vi "RSZVB Set Trace Format ZVR.vi"(8 "error in (no error)":errorcluster {"code" format="%.0x"}, 10 "Data Format (0: Unformatted)":i32(ring) items=["Unformatted", "Formatted", "Unformatted With Trace Mathematics"], 11 "VISA session":refnum<visa-resource-name>) -> (0 "error out":errorcluster {"code" format="%.0x"}, 3 "dup VISA session":refnum<visa-resource-name>)   [LabVIEW 2011]
doc: "This VI defines the format for traces retrieved with the ZVR-compatible command TRACe[:DATA][:RESPonse][:ALL]? \n\nNote(s):\n\n(1) This VI is ZVR compatible.\n\nRemote-control command(s):\nFORMat:DEXPort:SOURce FDATa | SDATa | MDATa"
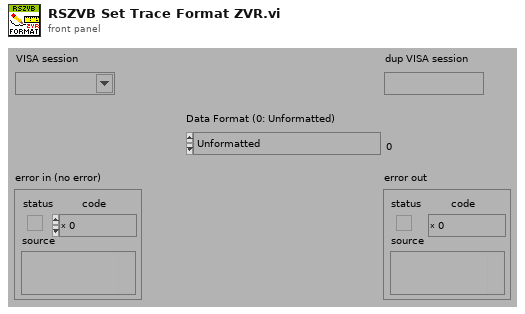
[diagram p1: front panel]
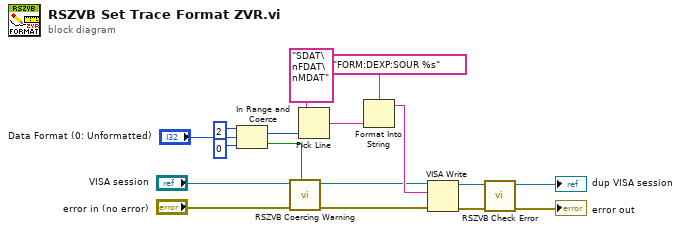
[diagram p0: block diagram]
diagram:
  n1 = In Range and Coerce(upper limit=2, x="Data Format (0: Unformatted)", lower limit=0) -> (coerced(x)=w14:i32, In Range?=w2:bool)
  n2 = call "RSZVB Coercing Warning.vi"("In Range?"=w2, "error in (no error)"="error in (no error)", "VISA session"="VISA session") -> ("error out"=w10:errorcluster, "dup VISA session"=w8:refnum<visa-resource-name>)  [unwired: 7 in]
  n3 = Pick Line(multi-line string="SDAT\nFDAT\nMDAT", line index=w14) -> (output string=w1:string)  [unwired: 1 in]
  n4 = Format Into String(format string="FORM:DEXP:SOUR %s", w1) -> (resulting string=w9:string)  [unwired: 2 in, 1 out]
  n5 = VISA Write(VISA resource name=w8, write buffer=w9, error in (no error)=w10) -> (VISA resource name out=w11:refnum<visa-resource-name>, error out=w12:errorcluster)  [unwired: 1 out]
  n6 = call "RSZVB Check Error.vi"("error in (no error)"=w12, "VISA session"=w11) -> ("error out"=→"error out":errorcluster, "dup VISA session"=→"dup VISA session":refnum<visa-resource-name>)  [unwired: 8 in]
